vi "GettingSerialDataG.vi"() -> ()   [LabVIEW 2020]
uses:
  State2.ctl
  Data2.ctl
  <vilib>/Instr/_visa.llb/VISA Configure Serial Port (Instr).vi
  <vilib>/Utility/file.llb/Write Delimited Spreadsheet (DBL).vi
panel:
  out "State2":T1=enum."ReadSerial"
  in  "Save Button":bool
  in  "Rec Button":bool
  in  "VISA resource name (COM)":refnum<visa-resource-name>="CNCB0"
  out "Temperature Graph":T2(graph)
  in  "stop":bool
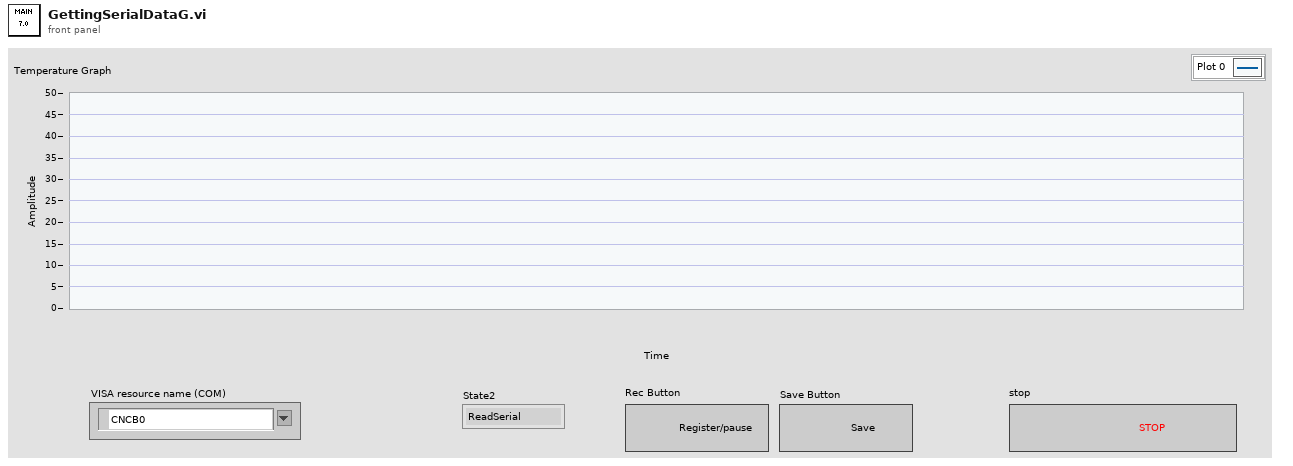
[diagram p1: front panel]
types:
  T1 = typedef "State2.ctl" = enum16{"Initialize", "ReadSerial", "ShowData", "SaveData", "Finalize"}
  T2 = cluster{"seconds since 1Jan1904":timestamp, dbl, dbl}[]
  T3 = enum8{"Enabled", "Disabled", "Disabled and Grayed Out"}
  T4 = enum16{"open", "replace", "create", "open or create", "replace or create", "replace or create with confirmation"}
  T5 = typedef "Data2.ctl" = cluster{"time":timestamp, "Temperature":dbl, "Viscosity":dbl}
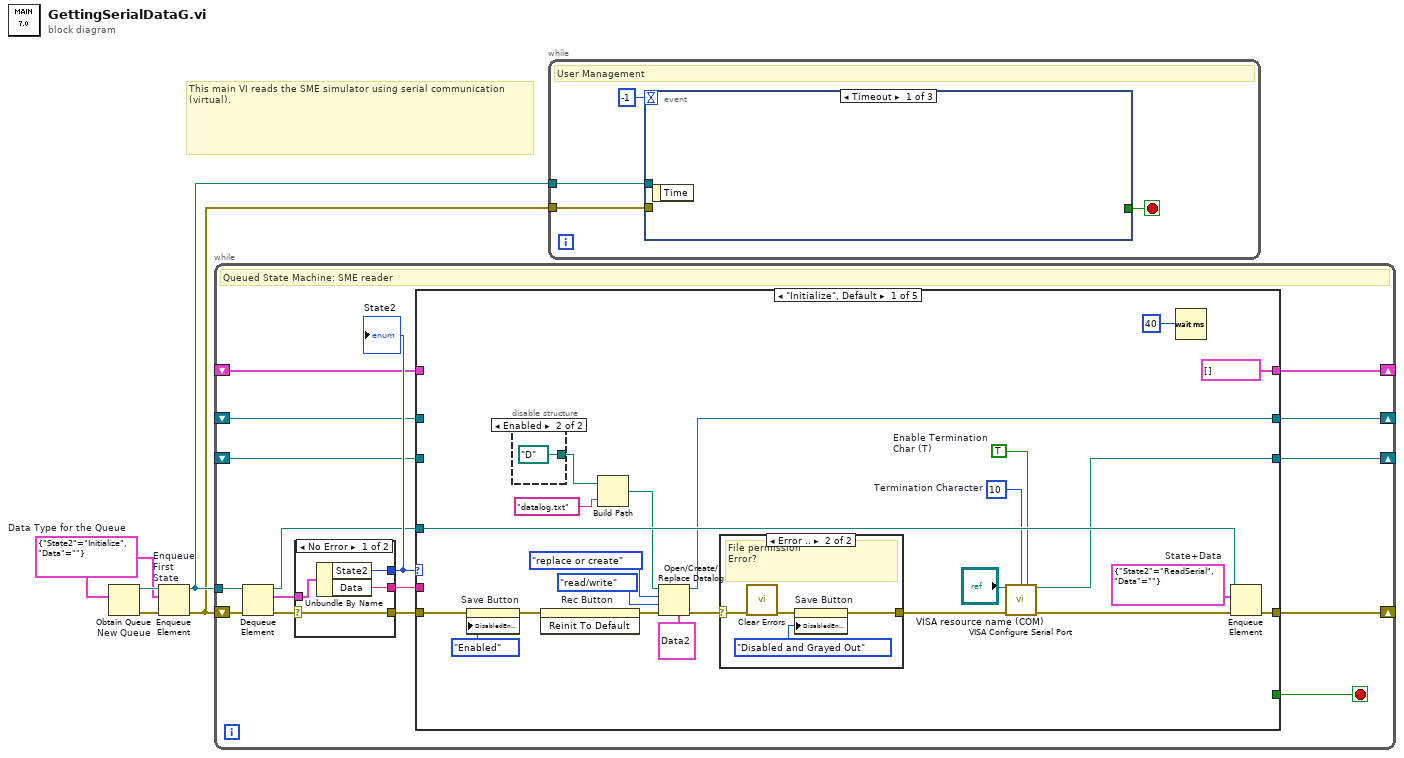
[diagram p0: block diagram]
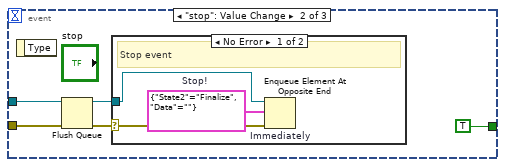
[diagram p2: hidden frame]
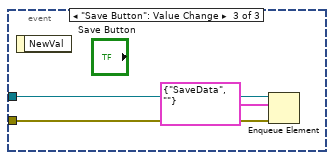
[diagram p4: hidden frame]
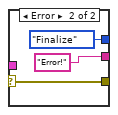
[diagram p5: hidden frame]
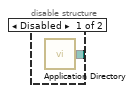
[diagram p6: hidden frame]
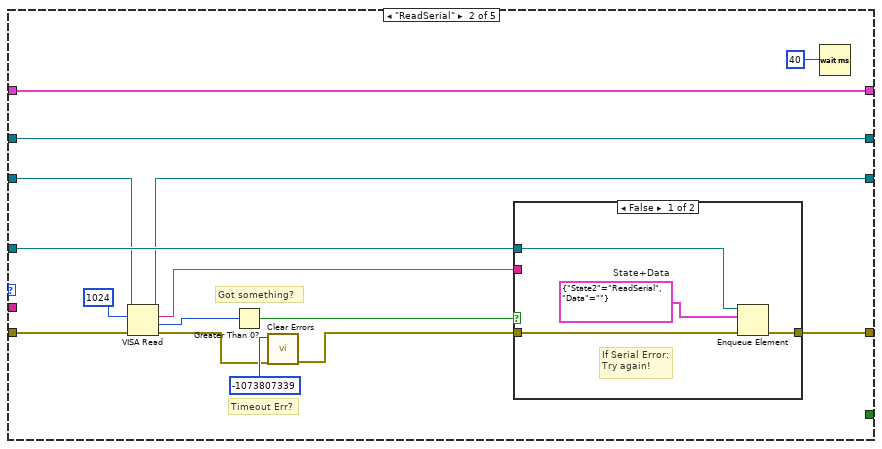
[diagram p8: hidden frame]
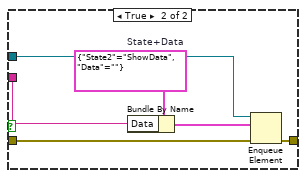
[diagram p9: hidden frame]
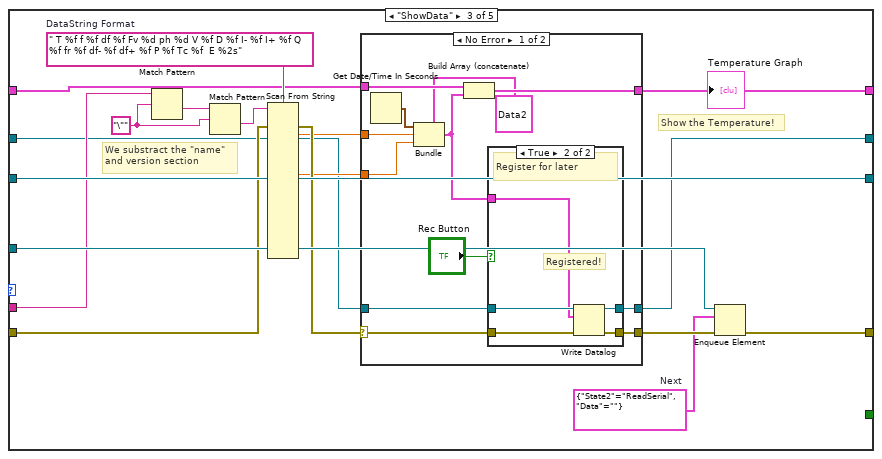
[diagram p10: hidden frame]
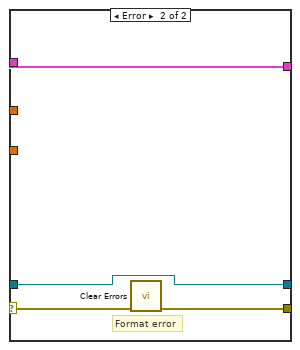
[diagram p12: hidden frame]
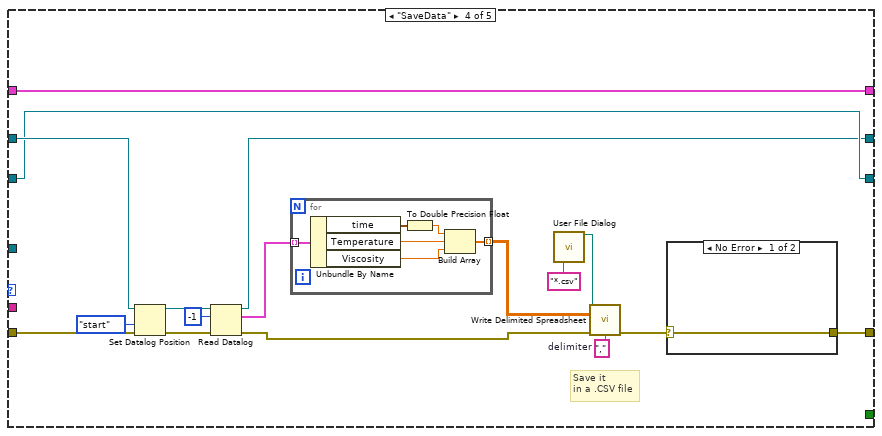
[diagram p13: hidden frame]
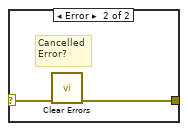
[diagram p14: hidden frame]
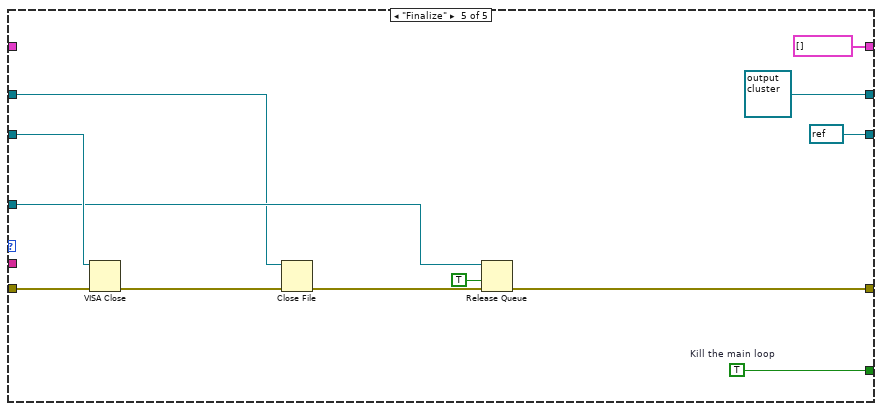
[diagram p15: hidden frame]
diagram:
  w4 = cluster{"State2":T1, "Data":string} {"State2"=enum."Initialize", "Data"=""}  # Data Type for the Queue
  # "This main VI reads the SME simulator using serial communication (virtual)."
  n1 = Obtain Queue "New Queue"(element data type=w4) -> (queue out=w5:refnum<queue>, error out=w3:errorcluster)  [unwired: 4 in, 1 out]
  n2 = Enqueue Element "Enqueue\nFirst\nState"(queue=w5, element=w4, error in (no error)=w3) -> (queue out=w2:refnum<queue>, error out=w1:errorcluster)  [unwired: 1 in, 1 out]
  n3 = while {
    shift-right: [w18] -> _
    shift-left: w1 -> [w14]
    shift-right: [w17] -> _
    shift-left: _ -> [w16]
    tunnel: w2 -> [w15]
    shift-right: [w8] -> _
    shift-left: _ -> [w9]
    shift-right: [w7] -> _
    shift-left: _ -> [w6]
    stop <- w11 stop-if-true
    # "Queued State Machine: SME reader"
    n4 = Dequeue Element(queue=w15, error in (no error)=w14) -> (queue out=w10:refnum<queue>, element=w12:cluster{"State2":T1, "Data":string}, error out=w13:errorcluster)  [unwired: 1 in, 1 out]
    n5 = case shown="No Error" w13 {
      selector: w13 -> [w22 w27]
      tunnel: w12 -> [w25 _]
      tunnel: [w24 State2."Finalize" ("State2")] -> w21
      tunnel: [w23 "Error!" ("Data")] -> w20
      tunnel: [w22 w27] -> w19
      frame No Error {
        n6 = Unbundle By Name(w25) -> ("State2"=w24:T1, "Data"=w23:string)
      }
      frame Error {
      }
    }
    "State2" <- w21
    n7 = case shown="\"Initialize\", Default" w21 {
      tunnel: w20 -> [_ _ w86 _ _]
      tunnel: w19 -> [w31 w66 w93 w140 w161]
      tunnel: [w50 w72 w99 w130 w158] -> w18
      tunnel: [w46 w64 w101 w127 refnum<visa-resource-name> refnum ("VISA resource name")] -> w17
      tunnel: w16 -> [_ w67 w101 w127 w162]
      tunnel: [_ _ _ _ w159] -> w11
      tunnel: w10 -> [w51 w73 w100 _ w157]
      tunnel: w9 -> [_ w71 w88 w141 _]
      tunnel: [T2 [] w71 w89 w141 T2 []] -> w8
      tunnel: [w39 w59 w84 w126 refnum<k1> refnum] -> w7
      tunnel: w6 -> [_ w59 w85 w129 w153]
      frame "Initialize", Default {
        w44 = cluster{"State2":T1, "Data":string} {"State2"=enum."ReadSerial", "Data"=""}  # State+Data
        w48 = u8 10  # Termination Character
        w49 = TRUE  # Enable Termination Char (T)
        n8 = property on="Save Button" class="Bool"(error in=w31, "DisabledEnum"=T3."Enabled" ("Disabled")) -> (error out=w30:errorcluster)  [unwired: 1 in, 1 out]
        n9 = disable-structure shown="Enabled" {
          disable-tunnel: [w52 path "D:/" ("Application Directory")] -> w42
          frame Disabled {
            n10 = call <vilib>:"Application Directory.vi"() -> ("Application Directory"=w52:path)
          }
          frame Enabled {
          }
        }
        n11 = invoke on="Rec Button" class="Bool (strict)" method="Reinit To Default"(error in=w30) -> (error out=w29:errorcluster)  [unwired: 2 in, 2 out]
        n12 = Build Path(base path=w42, name or relative path="datalog.txt") -> (appended path=w40:path)
        n13 = Open/Create/Replace Datalog(5:T5 {"time"=timestamp(0 s since 1904-01-01), "Temperature"=0.0, "Viscosity"=0.0} ("output cluster"), 8:w29, 9:enum16{"read/write", "read-only", "write-only"}."read/write" ("access (0:read/write)"), 10:T4."replace or create" ("operation (0:open)"), 11:w40) -> (0:w36:errorcluster, 3:w39:refnum<k1>)  [unwired: 1 in, 1 out]
        n14 = case shown="Error .." w36 {
          selector: w36 -> [w54 w58]
          tunnel: [w54 w56] -> w35
          frame No Error {
          }
          frame Error {
            # "File permission\nError?"
            n15 = call <vilib>:"Clear Errors.vi"("error in (no error)"=w58) -> ("error out"=w57:errorcluster)  [unwired: 5 in, 1 out]
            n16 = property on="Save Button" class="Bool"(error in=w57, "DisabledEnum"=T3."Disabled and Grayed Out" ("Disabled")) -> (error out=w56:errorcluster)  [unwired: 1 in, 1 out]
          }
        }
        n17 = call-poly "VISA Configure Serial Port"("VISA resource name"="VISA resource name (COM)", "termination char\n(0xA = '\\n' = LF)"=w48, "Enable Termination\nChar (T)"=w49, "error in (no error)"=w35) -> ("VISA resource name out"=w46:refnum<visa-resource-name>, "error out"=w45:errorcluster)  [unwired: 10 in]
        n18 = Wait (ms)(milliseconds to wait=u32 40) -> ()  [unwired: 1 out]
        n19 = Enqueue Element(queue=w51, element=w44, error in (no error)=w45) -> (error out=w50:errorcluster)  [unwired: 1 in, 2 out]
      }
      frame "ReadSerial" {
        # "Timeout Err?"
        # "Got something?"
        n20 = VISA Read(VISA resource name=w67, byte count=u32 1024, error in (no error)=w66) -> (VISA resource name out=w64:refnum<visa-resource-name>, read buffer=w63:string, return count=w68:u32, error out=w61:errorcluster)
        n21 = Greater Than 0?(x=w68) -> (x > 0?=w65:bool)
        n22 = call <vilib>:"Clear Errors.vi"("error in (no error)"=w61, "specific error code to clear (0: all)"=-1073807339 ("y")) -> ("error out"=w60:errorcluster)  [unwired: 4 in, 1 out]
        n23 = case shown="False" w65 {
          tunnel: w73 -> [w77 w83]
          tunnel: [w76 w82] -> w72
          tunnel: w60 -> [w74 w81]
          tunnel: w63 -> [_ w79]
          frame False {
            w75 = cluster{"State2":T1, "Data":string} {"State2"=enum."ReadSerial", "Data"=""}  # State+Data
            # "If Serial Error:\nTry again!"
            n24 = Enqueue Element(queue=w77, element=w75, error in (no error)=w74) -> (error out=w76:errorcluster)  [unwired: 1 in, 2 out]
          }
          frame True {
            w80 = cluster{"State2":T1, "Data":string} {"State2"=enum."ShowData", "Data"=""}  # State+Data
            n25 = Bundle By Name(cluster=w80, "Data"=w79) -> (w78:cluster{"State2":T1, "Data":string})
            n26 = Enqueue Element(queue=w83, element=w78, error in (no error)=w81) -> (error out=w82:errorcluster)  [unwired: 1 in, 2 out]
          }
        }
        n27 = Wait (ms)(milliseconds to wait=u32 40) -> ()  [unwired: 1 out]
      }
      frame "ShowData" {
        w91 = cluster{"State2":T1, "Data":string} {"State2"=enum."ReadSerial", "Data"=""}  # Next
        w96 = "\"" ("regular expression")
        w94 = " T %f f %f df %f Fv %d ph %d V %f D %f I- %f I+ %f Q %f fr %f df- %f df+ %f P %f Tc %f  E %2s"  # DataString Format
        # "We substract the \"name\"\nand version section"
        # "Show the Temperature!"
        n28 = Match Pattern(string=w86, regular expression=w96) -> (after substring=w97:string)  [unwired: 1 in, 3 out]
        n29 = Match Pattern(string=w97, regular expression=w96) -> (after substring=w95:string)  [unwired: 1 in, 3 out]
        n30 = Scan From String(format string=w94, input string=w95, error in=w93) -> (error out=w92:errorcluster, output 1=w90:dbl, output 6=w87:dbl)  [unwired: 31 in, 2 out]
        n31 = case shown="No Error" w92 {
          selector: w92 -> [w108 w124]
          tunnel: [w105 w123] -> w98
          tunnel: w88 -> [w112 w122]
          tunnel: w90 -> [w110 _]
          tunnel: [w113 w122] -> w89
          tunnel: w87 -> [w109 _]
          tunnel: w85 -> [w107 w121]
          tunnel: [w106 w121] -> w84
          frame No Error {
            n32 = Get Date/Time In Seconds() -> (seconds since 1Jan1904=w111:timestamp)
            n33 = Bundle(cluster=T5 {"time"=timestamp(0 s since 1904-01-01), "Temperature"=0.0, "Viscosity"=0.0} ("output cluster"), "time"=w111, "Temperature"=w110, "Viscosity"=w109) -> (w102:T5)
            n34 = Build Array (concatenate)(w112, w102) -> (w113:T5[])
            n35 = case shown="True" "Rec Button" {
              tunnel: w108 -> [w114 w120]
              tunnel: w107 -> [w115 w119]
              tunnel: [w115 w118] -> w106
              tunnel: [w114 w117] -> w105
              tunnel: w102 -> [_ w116]
              frame False {
                # "Pause or \nhasn't started"
              }
              frame True {
                # "Registered!"
                # "Register for later"
                n36 = Write Datalog(4:w120, 6:w116, 7:w119) -> (0:w117:errorcluster, 3:w118:refnum<k1>)
              }
            }
          }
          frame Error {
            # "Format error"
            n37 = call <vilib>:"Clear Errors.vi"("error in (no error)"=w124) -> ("error out"=w123:errorcluster)  [unwired: 5 in, 1 out]
          }
        }
        "Temperature Graph" <- w89
        n38 = Enqueue Element(queue=w100, element=w91, error in (no error)=w98) -> (error out=w99:errorcluster)  [unwired: 1 in, 2 out]
      }
      frame "SaveData" {
        w125 = ","  # delimiter
        # "Save it\nin a .CSV file"
        n39 = Set Datalog Position(4:w140, 5:enum16{"start", "end", "current"}."start" ("from (0:start)"), 7:w129) -> (0:w137:errorcluster, 3:w138:refnum<k1>)  [unwired: 1 in]
        n40 = Read Datalog(4:w137, 6:-1 ("count (1)"), 7:w138) -> (0:w132:errorcluster, 2:w136:T5[], 3:w126:refnum<k1>)
        n41 = for {
          tunnel: w136 -> [w150] mode=indexing
          tunnel: [w145] -> w135 mode=indexing
          n42 = Unbundle By Name(w150) -> ("time"=w147:timestamp, "Temperature"=w148:dbl, "Viscosity"=w149:dbl)
          n43 = To Double Precision Float(number=w147) -> (double precision float=w146:dbl)
          n44 = Build Array(w146, w148, w149) -> (w145:dbl[])
        }
        n45 = call "User File Dialog"("pattern (all files)"="*.csv") -> ("selected path"=w133:path)  [unwired: 11 in, 3 out]
        n46 = call-poly <vilib>:"Write Delimited Spreadsheet.vi"("file path (dialog if empty)"=w133, "2D data"=w135, "error in (no error)"=w132, "delimiter (\\t)"=w125) -> ("error out"=w131:errorcluster)  [unwired: 10 in, 1 out]
        n47 = case shown="No Error" w131 {
          selector: w131 -> [w142 w144]
          tunnel: [w142 w143] -> w130
          frame No Error {
          }
          frame Error {
            # "Cancelled\nError?"
            n48 = call <vilib>:"Clear Errors.vi"("error in (no error)"=w144) -> ("error out"=w143:errorcluster)  [unwired: 5 in, 1 out]
          }
        }
      }
      frame "Finalize" {
        w159 = TRUE  # Kill the main loop
        n49 = VISA Close(VISA resource name=w162, error in (no error)=w161) -> (error out=w152:errorcluster)
        n50 = Close File(refnum=w153, error in=w152) -> (error out=w151:errorcluster)  [unwired: 1 out]
        n51 = Release Queue(queue=w157, force destroy? (F)=TRUE, error in (no error)=w151) -> (error out=w158:errorcluster)  [unwired: 2 out]
      }
    }
  }
  n52 = while {
    tunnel: w2 -> [w164]
    tunnel: w1 -> [w163]
    stop <- w165 stop-if-true
    # "User Management"
    n53 = event shown="[0] Timeout" {
      selector: _ -> [_ _ _]
      dyn-events: _ -> [_ _ _]
      timeout: -1 -> [_ _ _]
      tunnel: [_ TRUE _] -> w165
      tunnel: w164 -> [_ w169 w177]
      tunnel: w163 -> [_ w170 w175]
      event Timeout {
        n54 = event-data() -> ()  [unwired: 1 in, 1 out]
      }
      event "stop": Value Change {
        n55 = event-data() -> ()  [unwired: 1 in, 1 out]
        n56 = Flush Queue(queue=w169, error in (no error)=w170) -> (queue out=w168:refnum<queue>, error out=w167:errorcluster)  [unwired: 1 out]
        n57 = case shown="No Error" w167 {
          selector: w167 -> [w173 _]
          tunnel: w168 -> [w174 _]
          frame No Error {
            w172 = cluster{"State2":T1, "Data":string} {"State2"=enum."Finalize", "Data"=""}  # Stop!
            # "Stop event"
            n58 = Enqueue Element At Opposite End "Immediately"(queue=w174, element=w172, error in (no error)=w173) -> ()  [unwired: 1 in, 3 out]
          }
          frame Error {
            # "Already dead"
          }
        }
      }
      event "Save Button": Value Change {
        n59 = event-data() -> ()  [unwired: 1 in, 1 out]
        n60 = Enqueue Element(queue=w177, element=cluster{"State2":T1, "Data":string} {"State2"=enum."SaveData", "Data"=""}, error in (no error)=w175) -> ()  [unwired: 1 in, 3 out]
      }
    }
  }
